vi "string conversion.vi"() -> ()   [LabVIEW 2017]
panel:
  out "Array":string[](array[string])
  out "String 2":string
  out "String":string="5314216\n21102024010011\nA1105000100"
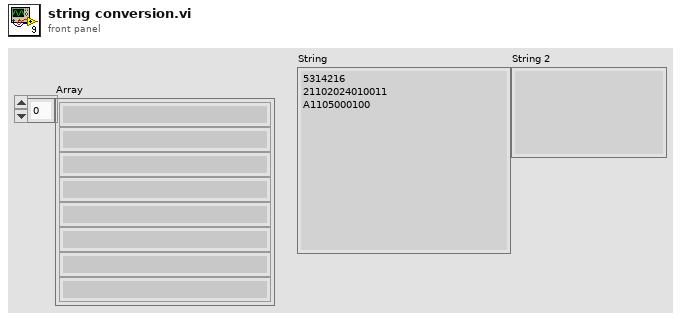
[diagram p1: front panel]
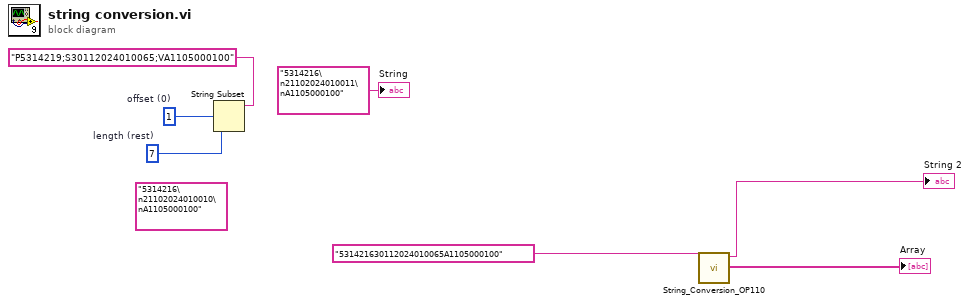
[diagram p0: block diagram]
diagram:
  w5 = 7  # length (rest)
  w6 = 1  # offset (0)
  (unwired) "5314216\n21102024010010\nA1105000100"
  n1 = String Subset(string="P5314219;S30112024010065;VA1105000100", offset (0)=w6, length (rest)=w5) -> ()  [unwired: 1 out]
  n2 = call "String_Conversion_OP110.vi"("String in"="531421630112024010065A1105000100") -> ("Array"=→"Array":string[], "String out"=→"String 2":string)  [unwired: 9 in]
  "String" <- "5314216\n21102024010011\nA1105000100"
